vi "readyQueues.vi"(8 "error in (no error)":errorcluster) -> (0 "error out":errorcluster, 3 "Queues":T1)   [LabVIEW 2010]
uses:
  internal_queues.ctl
  line_info.ctl
  volume_with_lines.ctl
  volume_info.ctl
  kalman_result_scaled.ctl
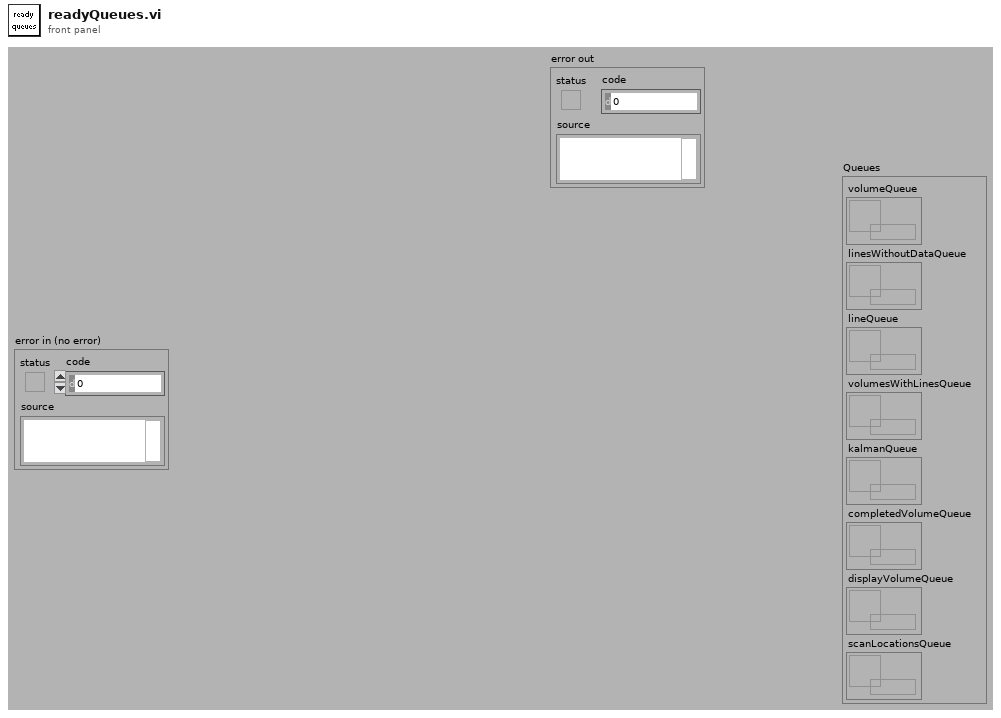
[diagram p1: front panel]
types:
  T1 = typedef "internal_queues.ctl" = cluster{"volumeQueue":refnum<queue>, "linesWithoutDataQueue":refnum<queue>, "lineQueue":refnum<queue>, "volumesWithLinesQueue":refnum<queue>, "kalmanQueue":refnum<queue>, "completedVolumeQueue":refnum<queue>, "displayVolumeQueue":refnum<queue>, "scanLocationsQueue":refnum<queue>}
  T2 = typedef "kalman_result_scaled.ctl" = cluster{"axis":u8, "pos":dbl, "vel":dbl, "p_err":dbl, "v_err":dbl, "n photon ch 0":u32, "n photon ch 1":u32, "elapsed time":dbl}
  T3 = typedef "volume_with_lines.ctl" = cluster{"volume info":T4, "lines":T5[]}
  T4 = typedef "volume_info.ctl" = cluster{"min x":i16, "deltaX":dbl, "num x":u32, "max x":i16, "min y":i16, "deltaY":dbl, "num y":u32, "max y":i16, "num z":u32, "num voxels":u32, "voxels read":u32, "volume num":u32}
  T5 = typedef "line_info.ctl" = cluster{"start X":i16, "start Y":i16, "start Z":i16, "end X":i16, "end Y":i16, "end Z":i16, "num z":u8, "voxel data":u32[], "volume num":u32, "line number":u16, "unused":u16}
  T6 = cluster{"ch0 volume":u32[][][], "ch1 volume":u32[][][], "ff 0+1":u32[][][], "fb 0+1":u32[][][]}
  T7 = cluster{"volume info":cluster{"min x":i16, "deltaX":dbl, "num x":u32, "max x":i16, "min y":i16, "deltaY":dbl, "num y":u32, "max y":i16, "num z":u32, "num voxels":u32, "voxels read":u32, "volume num":u32}, "buffer":u32[]}
  T8 = cluster{"min x":i16, "deltaX":dbl, "num x":u32, "max x":i16, "min y":i16, "deltaY":dbl, "num y":u32, "max y":i16, "num z":u32, "num voxels":u32, "voxels read":u32, "volume num":u32}
  T9 = cluster{"queue out":refnum<queue>, "queue out":refnum<queue>, "queue out":refnum<queue>, "queue out":refnum<queue>, "queue out":refnum<queue>, "queue out":refnum<queue>, "queue out":refnum<queue>, "queue out":refnum<queue>}
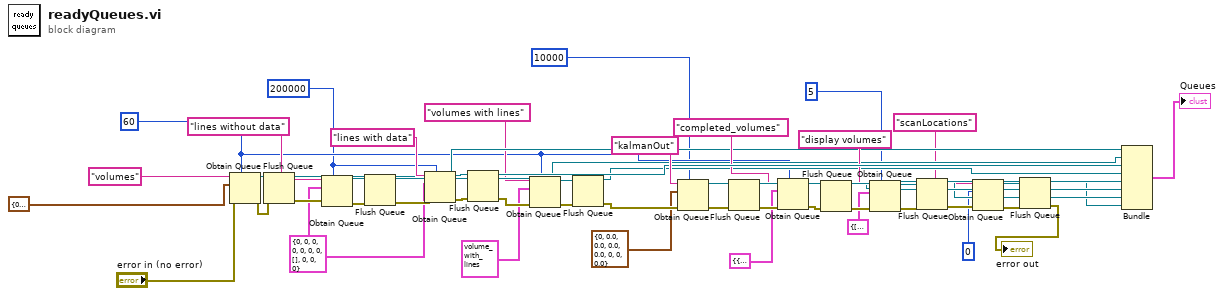
[diagram p0: block diagram]
diagram:
  w3 = 200000 ("max queue size (-1, unlimited)")
  w4 = 60 ("max queue size (-1, unlimited)")
  w23 = T5 {"start X"=0, "start Y"=0, "start Z"=0, "end X"=0, "end Y"=0, "end Z"=0, "num z"=0, "voxel data"=[], "volume num"=0, "line number"=0, "unused"=0} ("line status")
  n1 = Obtain Queue(max queue size (-1, unlimited)=w4, name (unnamed)="volumes" ("volumes"), element data type=T8 {"min x"=0, "deltaX"=0.0, "num x"=0, "max x"=0, "min y"=0, "deltaY"=0.0, "num y"=0, "max y"=0, "num z"=0, "num voxels"=0, "voxels read"=0, "volume num"=0} ("volume info"), error in (no error)="error in (no error)") -> (queue out=w48:refnum<queue>, error out=w45:errorcluster)  [unwired: 1 in, 1 out]
  n2 = Flush Queue(queue=w48, error in (no error)=w45) -> (queue out=w26:refnum<queue>, error out=w28:errorcluster)  [unwired: 1 out]
  n3 = Obtain Queue(max queue size (-1, unlimited)=w3, name (unnamed)="lines without data", element data type=w23, error in (no error)=w28) -> (queue out=w24:refnum<queue>, error out=w27:errorcluster)  [unwired: 1 in, 1 out]
  n4 = Flush Queue(queue=w24, error in (no error)=w27) -> (queue out=w21:refnum<queue>, error out=w25:errorcluster)  [unwired: 1 out]
  n5 = Obtain Queue(max queue size (-1, unlimited)=w3, name (unnamed)="lines with data", element data type=w23, error in (no error)=w25) -> (queue out=w47:refnum<queue>, error out=w43:errorcluster)  [unwired: 1 in, 1 out]
  n6 = Flush Queue(queue=w47, error in (no error)=w43) -> (queue out=w44:refnum<queue>, error out=w17:errorcluster)  [unwired: 1 out]
  n7 = Obtain Queue(max queue size (-1, unlimited)=w4, name (unnamed)="volumes with lines", element data type=T3 {"volume info"={"min x"=0, "deltaX"=0.0, "num x"=0, "max x"=0, "min y"=0, "deltaY"=0.0, "num y"=0, "max y"=0, "num z"=0, "num voxels"=0, "voxels read"=0, "volume num"=0}, "lines"=[]} ("Cluster"), error in (no error)=w17) -> (queue out=w19:refnum<queue>, error out=w18:errorcluster)  [unwired: 1 in, 1 out]
  n8 = Flush Queue(queue=w19, error in (no error)=w18) -> (queue out=w13:refnum<queue>, error out=w16:errorcluster)  [unwired: 1 out]
  n9 = Obtain Queue(max queue size (-1, unlimited)=10000, name (unnamed)="kalmanOut", element data type=T2 {"axis"=0, "pos"=0.0, "vel"=0.0, "p_err"=0.0, "v_err"=0.0, "n photon ch 0"=0, "n photon ch 1"=0, "elapsed time"=0.0} ("kalman result"), error in (no error)=w16) -> (queue out=w46:refnum<queue>, error out=w41:errorcluster)  [unwired: 1 in, 1 out]
  n10 = Flush Queue(queue=w46, error in (no error)=w41) -> (queue out=w42:refnum<queue>, error out=w40:errorcluster)  [unwired: 1 out]
  n11 = Obtain Queue(max queue size (-1, unlimited)=w4, name (unnamed)="completed_volumes", element data type=T7 {"volume info"={"min x"=0, "deltaX"=0.0, "num x"=0, "max x"=0, "min y"=0, "deltaY"=0.0, "num y"=0, "max y"=0, "num z"=0, "num voxels"=0, "voxels read"=0, "volume num"=0}, "buffer"=[]} ("completed volumes"), error in (no error)=w40) -> (queue out=w38:refnum<queue>, error out=w39:errorcluster)  [unwired: 1 in, 1 out]
  n12 = Flush Queue(queue=w38, error in (no error)=w39) -> (queue out=w35:refnum<queue>, error out=w34:errorcluster)  [unwired: 1 out]
  n13 = Obtain Queue(max queue size (-1, unlimited)=5, name (unnamed)="display volumes", element data type=T6 {"ch0 volume"=[], "ch1 volume"=[], "ff 0+1"=[], "fb 0+1"=[]} ("volumes for display"), error in (no error)=w34) -> (queue out=w30:refnum<queue>, error out=w33:errorcluster)  [unwired: 1 in, 1 out]
  n14 = Flush Queue(queue=w30, error in (no error)=w33) -> (queue out=w29:refnum<queue>, error out=w12:errorcluster)  [unwired: 1 out]
  n15 = Obtain Queue(name (unnamed)="scanLocations", element data type=u32 0, error in (no error)=w12) -> (queue out=w9:refnum<queue>, error out=w11:errorcluster)  [unwired: 2 in, 1 out]
  n16 = Flush Queue(queue=w9, error in (no error)=w11) -> (queue out=w6:refnum<queue>, error out=→"error out":errorcluster)  [unwired: 1 out]
  n17 = Bundle("queue out"=w26, "queue out"=w21, "queue out"=w44, "queue out"=w13, "queue out"=w42, "queue out"=w35, "queue out"=w29, "queue out"=w6) -> (→"Queues":T9)  [unwired: 1 in]
